vi "BAP4B.vi"() -> ()   [LabVIEW 2014]
doc: "BAP4B\n\nSimulates a four way traffic intersection with the following settings:\n\nAll On: used to test the functionality of the lights themselves, and in this case all lights are on.\nBlinking: used when the light malfunctions and the traffic operates as instead as four way stop sign. The \"don't walk\" and stop lights turn on and off.\nAutomatic: used as a functioning four way traffic intersection. Lights transition from \"caution,\" \"go's,\" \"stops,\" and \"left turns\" as well as indicating when to walk. \n\nBeverly Abadines\nPHY 350\nP4"
uses:
  typedefs/stop light.ctl
  typedefs/left arrow.ctl
  typedefs/walk light.ctl
  typedefs/control mode enum.ctl
  typedefs/system state cluster.ctl
  typedefs/state enum.ctl
panel:
  out "system state":T1={"last light state"=enum."init", "light state"=enum."init", "state time (ms)"=10000, "current time (ms)"=0, "time remaining (ms)"=0, "change state"=FALSE}
  in  "mode set":T3
  in  "exit":bool
  out "WS walk":T4
  out "WN walk":T4
  out "ES walk":T4
  out "EN walk":T4
  out "SE walk":T4=TRUE
  out "SW walk":T4=TRUE
  out "NE walk":T4=TRUE
  out "NW walk":T4=TRUE
  out "East Light":T5={"stop"=FALSE, "caution"=FALSE, "go"=TRUE, "arrow"=FALSE}
  out "West Light":T5={"stop"=FALSE, "caution"=FALSE, "go"=TRUE, "arrow"=FALSE}
  out "North Light":T5={"stop"=TRUE, "caution"=FALSE, "go"=FALSE, "arrow"=FALSE}
  out "South Light":T5={"stop"=TRUE, "caution"=FALSE, "go"=FALSE, "arrow"=FALSE}
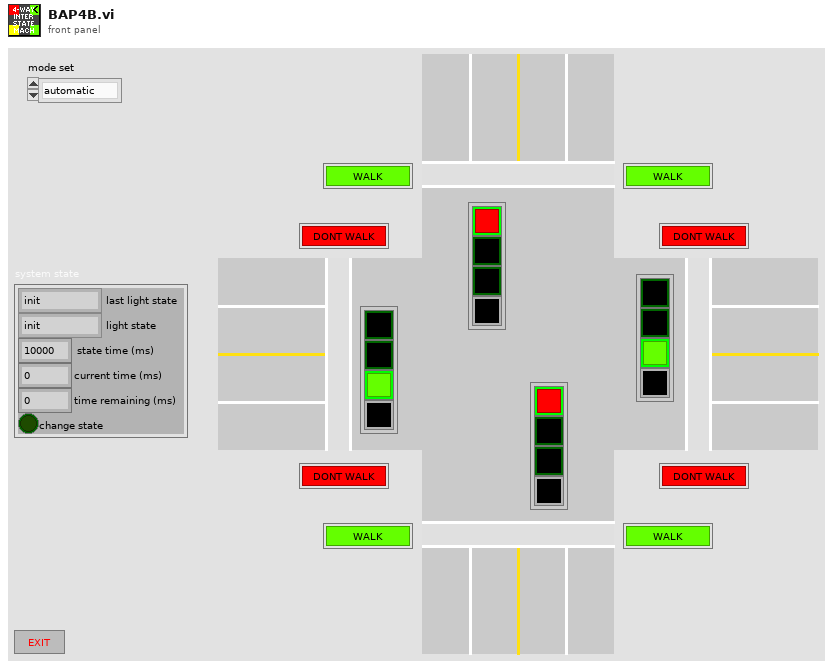
[diagram p1: front panel]
types:
  T1 = typedef "system state cluster.ctl" = cluster{"last light state":T2, "light state":T2, "state time (ms)":i32, "current time (ms)":i32, "time remaining (ms)":i32, "change state":bool}
  T2 = typedef "state enum.ctl" = enum16{"init", "idle", "left turn E", "go EW", "caution EW", "left turn W", "left turn N", "go NS", "caution NS", "left turn S", "blink on", "blink off", "all on test", "exit"}
  T3 = typedef "control mode enum.ctl" = enum16{"automatic", "blinking", "all on test"}
  T4 = typedef "walk light.ctl" = bool
  T5 = typedef "stop light.ctl" = cluster{"stop":bool, "caution":bool, "go":bool, "arrow":T6}
  T6 = typedef "left arrow.ctl" = bool
  T7 = typedef "all lights.ctl" = cluster{"east lights":T8, "west lights":T8, "north lights":T8, "south lights":T8}
  T8 = typedef "light set.ctl" = cluster{"light":T5, "walk A":T4, "walk B":T4}
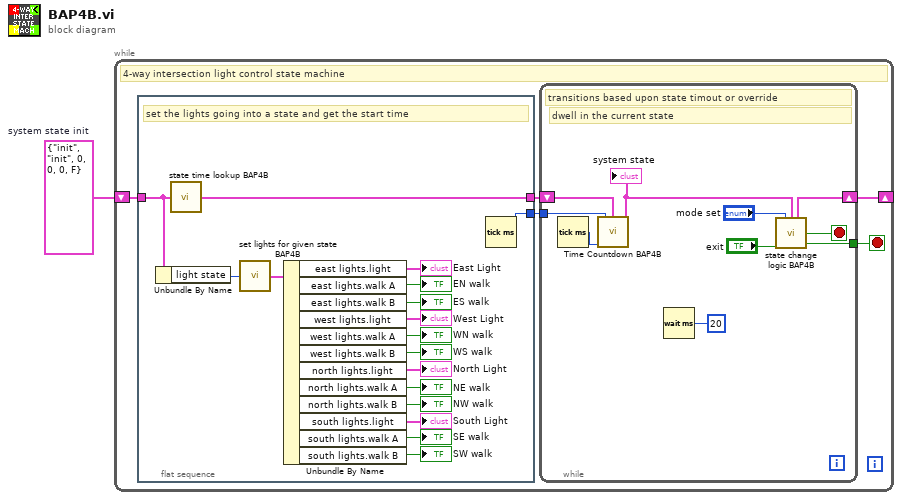
[diagram p0: block diagram]
diagram:
  w1 = T1 {"last light state"=enum."init", "light state"=enum."init", "state time (ms)"=0, "current time (ms)"=0, "time remaining (ms)"=0, "change state"=FALSE}  # system state init
  n1 = while {
    shift-right: [w4] -> _
    shift-left: w1 -> [w6]
    stop <- w2 stop-if-true
    # "4-way intersection light control state machine"
    n2 = flat-sequence {
      tunnel: w6 -> [w17]
      tunnel: [w18] -> w5
      tunnel: [w19] -> w3
      frame #0 {
        # "set the lights going into a state and get the start time"
        n3 = Unbundle By Name(w17) -> ("light state"=w21:T2)
        n4 = call "state time lookup BAP4B.vi"("system state in"=w17) -> ("system state out"=w18:T1)  [unwired: 14 in]
        n5 = call "set lights for given state BAP4B.vi"("light state"=w21) -> ("all lights out"=w20:T7)  [unwired: 14 in]
        n6 = Unbundle By Name(w20) -> ("east lights.light"=→"East Light":T5, "east lights.walk A"=→"EN walk":T4, "east lights.walk B"=→"ES walk":T4, "west lights.light"=→"West Light":T5, "west lights.walk A"=→"WN walk":T4, "west lights.walk B"=→"WS walk":T4, "north lights.light"=→"North Light":T5, "north lights.walk A"=→"NE walk":T4, "north lights.walk B"=→"NW walk":T4, "south lights.light"=→"South Light":T5, "south lights.walk A"=→"SE walk":T4, "south lights.walk B"=→"SW walk":T4)
        n7 = Tick Count (ms)() -> (millisecond timer value=w19:u32)
      }
    }
    n8 = while {
      shift-right: [w13] -> w4
      shift-left: w5 -> [w15]
      tunnel: [w14] -> w2
      tunnel: w3 -> [w8]
      stop <- w9 stop-if-true
      # "dwell in the current state"
      # "transitions based upon state timout or override"
      n9 = Tick Count (ms)() -> (millisecond timer value=w7:u32)
      n10 = call "Time Countdown BAP4B.vi"("Before Loop"=w8, "system state in"=w15, "After  Loop"=w7) -> ("system state out"=w12:T1)  [unwired: 5 in, 1 out]
      "system state" <- w12
      n11 = Wait (ms)(milliseconds to wait=u32 20) -> ()  [unwired: 1 out]
      n12 = call "state change logic BAP4B.vi"("mode set"="mode set", "system state in"=w12, "exit"="exit") -> ("system state out"=w13:T1, "change state"=w9:bool, "exit program"=w14:bool)  [unwired: 10 in]
    }
  }
